vi "new_portcullis.vi"(9 "Arm Down":bool, 10 "Arm Up":bool, 11 "Start Portcullis":bool) -> (1 "Done":bool, 2 "Arcade Drive":cluster{"x":dbl, "y":dbl}, 3 "Arm Solenoid":bool)   [LabVIEW 2015]
uses:
  new_portcullis_states.ctl
  Sensors.vi
panel:
  in  "Drive Thru Speed":dbl
  in  "Kd":dbl format="%#_13g"
  in  "Ki":dbl format="%#_13g"
  in  "Kp":dbl format="%#_13g"
  in  "up ramp tilt":dbl format="%#_13g"
  in  "Abort":bool
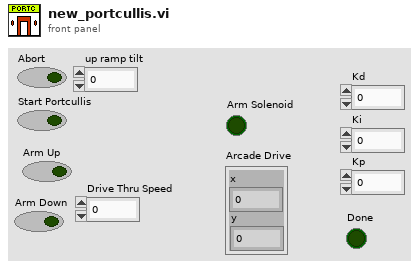
[diagram p1: front panel]
types:
  T1 = typedef "new_portcullis_states.ctl" = enum16{"Ready", "Arm Down", "Drive To Gate", "Raise Arm Driving", "Complete"}
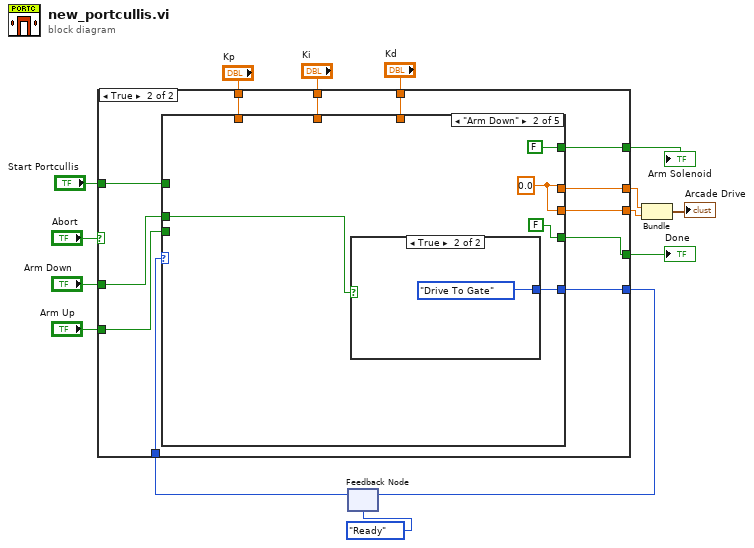
[diagram p0: block diagram]
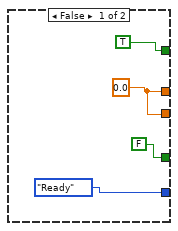
[diagram p2: hidden frame]
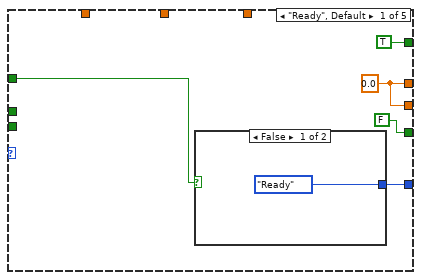
[diagram p3: hidden frame]
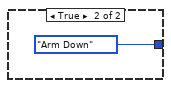
[diagram p4: hidden frame]
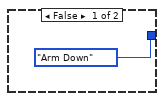
[diagram p5: hidden frame]
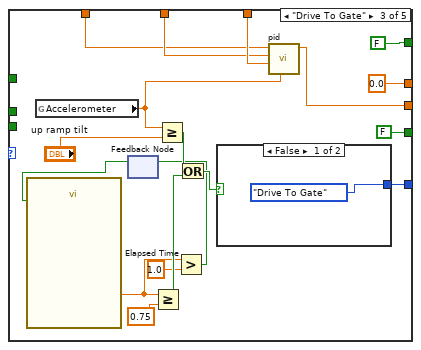
[diagram p6: hidden frame]
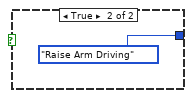
[diagram p7: hidden frame]
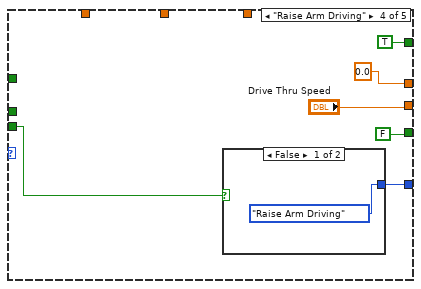
[diagram p8: hidden frame]
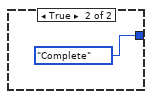
[diagram p9: hidden frame]
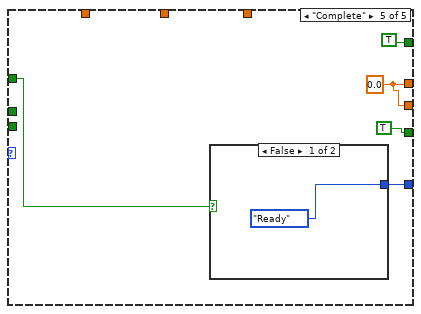
[diagram p10: hidden frame]
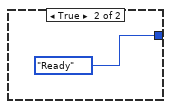
[diagram p11: hidden frame]
diagram:
  n1 = feedback #1(new_portcullis_states."Ready") -> (w14:T1)
  n2 = case shown="True" "Abort" {
    tunnel: w14 -> [_ w31]
    tunnel: [new_portcullis_states."Ready" w30] -> w12
    tunnel: [TRUE w29] -> w11
    tunnel: [w18 w28] -> w10
    tunnel: [w18 w27] -> w9
    tunnel: "Start Portcullis" -> [_ w26]
    tunnel: "Arm Down" -> [_ w25]
    tunnel: "Kd" -> [_ w24]
    tunnel: "Ki" -> [_ w23]
    tunnel: "Kp" -> [_ w22]
    tunnel: "Arm Up" -> [_ w21]
    tunnel: [FALSE w20] -> w1
    frame False {
      w18 = 0.0
    }
    frame True {
      n3 = case shown="\"Arm Down\"" w31 {
        tunnel: [w36 w41 w63 w71 w78] -> w30
        tunnel: [TRUE FALSE FALSE TRUE TRUE] -> w29
        tunnel: [w34 w42 0.0 0.0 w77] -> w28
        tunnel: [w34 w42 w57 "Drive Thru Speed" w77] -> w27
        tunnel: w26 -> [w33 _ _ _ w75]
        tunnel: w25 -> [_ w40 _ _ _]
        tunnel: w24 -> [_ _ w62 _ _]
        tunnel: w23 -> [_ _ w61 _ _]
        tunnel: w22 -> [_ _ w60 _ _]
        tunnel: w21 -> [_ _ _ w68 _]
        tunnel: [FALSE FALSE FALSE FALSE TRUE] -> w20
        frame "Ready", Default {
          w34 = 0.0
          n4 = case shown="False" w33 {
            tunnel: [new_portcullis_states."Ready" new_portcullis_states."Arm Down"] -> w36
            frame False {
            }
            frame True {
            }
          }
        }
        frame "Arm Down" {
          w42 = 0.0
          n5 = case shown="True" w40 {
            tunnel: [new_portcullis_states."Arm Down" new_portcullis_states."Drive To Gate"] -> w41
            frame False {
            }
            frame True {
            }
          }
        }
        frame "Drive To Gate" {
          n6 = global read "Sensors.vi" "Accelerometer"() -> (w58:dbl)
          n7 = feedback #2() -> (w47:bool)  [unwired: 1 in]
          n8 = call "Elapsed Time"("Reset"=w47) -> ("Elapsed Time (s)"=w49:dbl)  [unwired: 11 in, 7 out]
          n9 = Greater Or Equal?(x=w49, y=0.75) -> (x >= y?=w51:bool)
          n10 = Greater Or Equal?(x=w58, y="up ramp tilt") -> (x >= y?=w53:bool)
          n11 = Greater?(x=w49, y=1.0) -> (0:w48:bool)
          n12 = feedback-in #2(w48) -> ()
          n13 = Or(x=w53, y=w51) -> (x .or. y?=w54:bool)
          n14 = case shown="False" w54 {
            tunnel: [new_portcullis_states."Drive To Gate" new_portcullis_states."Raise Arm Driving"] -> w63
            frame False {
            }
            frame True {
            }
          }
          n15 = call "pid.vi"("y"=w58, "kd"=w62, "ki"=w61, "kp"=w60) -> ("Motor Command"=w57:dbl)  [unwired: 7 in]
        }
        frame "Raise Arm Driving" {
          n16 = case shown="False" w68 {
            tunnel: [new_portcullis_states."Raise Arm Driving" new_portcullis_states."Complete"] -> w71
            frame False {
            }
            frame True {
            }
          }
        }
        frame "Complete" {
          w77 = 0.0
          n17 = case shown="False" w75 {
            tunnel: [new_portcullis_states."Ready" new_portcullis_states."Ready"] -> w78
            frame False {
            }
            frame True {
            }
          }
        }
      }
    }
  }
  "Arm Solenoid" <- w11
  "Done" <- w1
  n18 = feedback-in #1(w12) -> ()
  n19 = Bundle(w10, "Drive Thru Speed"=w9) -> (→"Arcade Drive":cluster{dbl, "Drive Thru Speed":dbl})  [unwired: 1 in]
